vi "Main.vi"(11 "Module Admin":refnum<class "Delacor_lib_QMH_Module Admin.lvclass">) -> ()   [LabVIEW 2019, in "Main UI.lvlib"]
doc: "This template is based off of the Queued Message Handler design pattern and the Queued Message Handler project template that ships with LabVIEW.\n\nThe main difference is that the queue is private to this module and communication between modules is performed via Broadcast and Request events.\n\nRequest events are wrapped in public API methods and are handled in the Event Handling Loop (EHL) of this VI. Any module can register for Broadcast events sent by this module. The EHL generates messages based on user interface actions.\n\nThe Message Handling Loop (MHL) processes messages generated by the EHL, or by other messages. The messages are string values, so new messages can be added easily to the Message Cases case structure in the MHL. Each message cluster can also provide an optional value for Message Data, which is a variant that can be converted to whatever message-specific data is required.\n_____\nBased on Delacor QMH Project Template 4.0.0.47.\n_____\nBased on DQMH Project Template 6.1.0.94."
uses:
  Main UI.lvlib
  <vilib>/Delacor/Delacor QMH/Libraries/Module Admin_class/Delacor_lib_QMH_Module Admin.lvclass
  Main UI Shared/Decimation input --cluster.ctl
  Neo-Laura-LVOOP/Class Library/XYgraph_class/Units --enum.ctl
  Main UI Shared/Zpos type.ctl
  Main UI Shared/Apply_Savitsky--cluster.ctl
  FileReader/FPref_clustered--cluster references.ctl
  Main UI Shared/Boolean--FP cluster.ctl
  FileReader/FPref_cntrls--cluster references.ctl
  Main UI Shared/Indicators--FP cluster.ctl
  Module Data--cluster.ctl
  Neo-Laura-LVOOP/Class Library/XYgraph_class/XYgraph.lvclass
  <vilib>/Delacor/Delacor QMH/Libraries/Message Queue_class/Delacor_lib_QMH_Message Queue.lvclass/Delacor_lib_QMH_Message Queue.ctl
  <vilib>/event_ctls.llb/lveventtype.ctl
  Get analysis parameters Argument--cluster.ctl
  Get analysis parameters (Reply Payload)--cluster.ctl
  Stop Argument--cluster.ctl
  Filepath updated Argument--cluster.ctl
  Filepath Editor/Settings--cluster.ctl
  <vilib>/Delacor/Delacor QMH/Libraries/Module Admin_class/Delacor_lib_QMH_Module Admin.lvclass/Delacor_lib_QMH_Module Admin.ctl
  <vilib>/Delacor/Delacor QMH/Libraries/Message Queue_class/Delacor_lib_QMH_Enqueue Message (Single).vi
  <vilib>/Delacor/Delacor QMH/Libraries/Module Admin_class/Delacor_lib_QMH_Get External Launch.vi
  <vilib>/Utility/error.llb/Error Cluster From Error Code.vi
  <vilib>/ErrorRing/Error Ring.xnode
  <vilib>/Delacor/Delacor QMH/Libraries/Message Queue_class/Delacor_lib_QMH_Message Queue.lvclass
  Filepath Editor/Filepath Editor.lvlib
  Analysis/Analysis.lvlib
  FileReader/FileReader.lvlib
  Main UI Shared/MAIN UI Shared.lvlib
panel:
  out "XYgraph":cluster{"X":dbl[], "Y":dbl[]}[](graph)
  out "FileReader Running?":bool
  out "Settings Editor Running?":bool
  out "Analysis Running?":bool
  in  "Apply savitzky":T1
  in  "File number":i16=-21550 min=-1 max=1 step=1
  in  "Live?":bool
  in  "Z pos (ch)":T2 items=["Sensor FB", "Virtual"]
  in  "Tau Delay (ms)":dbl
  in  "Contact":T3={"Contact stat?"=TRUE, "Contact Spread of dev"=0.0} {"Contact Spread of dev" format="%#_13g"}
  out "Status":string
  in  "Y Units (micro)":T4="pico"
  in  "X Units (micro)":T4="micro"
  out "Files in Directory":i16=-21550
  out "Size (bytes)":i64=37399506 format="%.0p"
  in  "Savitzksky-Golay":T5={"Sidepoints (M)"=20.0, "Filter Order"=5} {"Filter Order" scale=0.0..10.0; "Sidepoints (M)" scale=0.0..10.0}
  out "Fcurve Metadata":string[][](table)
  in  "Decimation":T6={"App"={"Dec"=1, "apply"=FALSE}, "Con"={"Dec"=1, "apply"=FALSE}, "Ret"={"Dec"=1, "apply"=FALSE}}
  in  "Fwd":bool
  in  "Prev":bool
  in  "Settings":bool
  in  "Load":bool
  out "Filepath":path
  out "error out":errorcluster
  out "version":string
  # "TDMS file viewer"
  # "Def"
  # "Zpos"
  # "Contact"
  # "Analysis Parameters"
  # "Metadata"
  # "Decimation"
  # "Savitzsky-Golay Parameters"
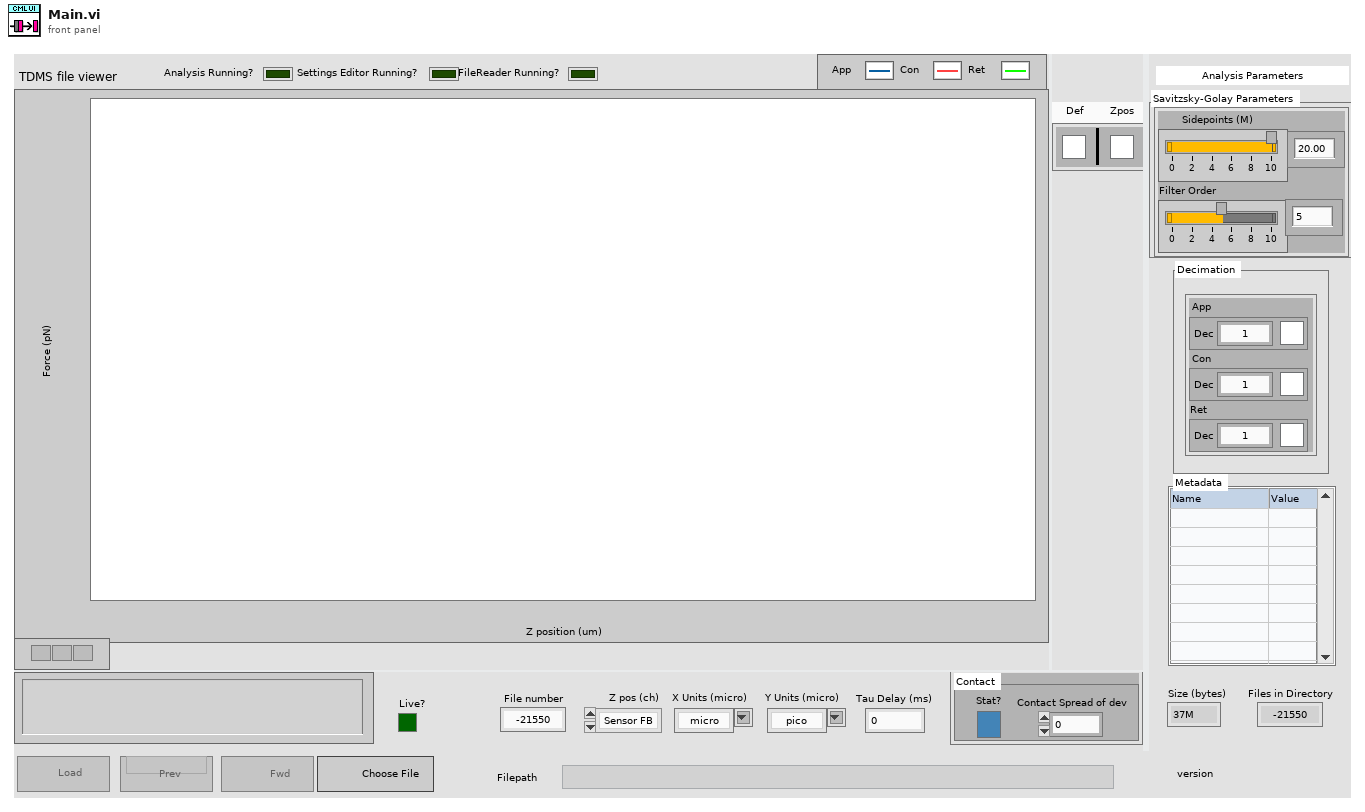
[diagram p1: front panel]
types:
  T1 = typedef "MAIN UI Shared.lvlib/Apply_Savitsky--cluster.ctl" = cluster{"Def":bool, "Zpos":bool}
  T2 = typedef "MAIN UI Shared.lvlib/Zpos type.ctl" = u16
  T3 = cluster{"Contact stat?":bool, "Contact Spread of dev":dbl}
  T4 = typedef "XYgraph.lvclass/Units --enum.ctl" = string
  T5 = cluster{"Sidepoints (M)":dbl, "Filter Order":i32}
  T6 = typedef "MAIN UI Shared.lvlib/Decimation input --cluster.ctl" = cluster{"App":cluster{"Dec":i32, "apply":bool}, "Con":cluster{"Dec":i32, "apply":bool}, "Ret":cluster{"Dec":i32, "apply":bool}}
  T7 = typedef "Indicators--FP cluster.ctl" = cluster{"Fcurve Metadata":refnum<vi>, "XYgraph":refnum<vi>, "Size (bytes)":refnum<vi>, "Files in Directory":refnum<vi>, "Filepath":refnum<vi>}
  T8 = typedef "FPref_clustered--cluster references.ctl" = cluster{" bools":T9, "cntrls":T10, "Ind":T7}
  T9 = typedef "MAIN UI Shared.lvlib/Boolean--FP cluster.ctl" = cluster{"Load":refnum<vi>, "Prev":refnum<vi>, "Fwd":refnum<vi>, "Set filepath":refnum<vi>}
  T10 = typedef "FPref_cntrls--cluster references.ctl" = cluster{"Z pos (ch)":refnum<vi>, "Tau Delay (ms)":refnum<vi>, "Y Units (micro)":refnum<vi>, "X Units (micro)":refnum<vi>, "Contact Spread of dev":refnum<vi>, "Contact stat?":refnum<vi>, "Decimation":refnum<vi>, "Savitzksky-Golay":refnum<vi>, "Apply savitzky ":refnum<vi>, "File number":refnum<vi>}
  T11 = cluster{"Fcurve Metadata":refnum<vi>, "XYgraph":refnum<vi>, "Size (bytes)":refnum<vi>, "Files in Directory":refnum<vi>, "Filepath":refnum<vi>}
  T12 = cluster{"Z pos (ch)":refnum<vi>, "Tau Delay (ms)":refnum<vi>, "Y Units (micro)":refnum<vi>, "X Units (micro)":refnum<vi>, "Contact Spread of dev":refnum<vi>, "Contact stat?":refnum<vi>, "Decimation":refnum<vi>, "Savitzksky-Golay":refnum<vi>, "Apply savitzky ":refnum<vi>, "File number":refnum<vi>}
  T13 = cluster{"Load":refnum<vi>, "Prev":refnum<vi>, "Fwd":refnum<vi>, "Set file path":refnum<vi>}
  T14 = typedef "Main UI.lvlib/Request Events--cluster.ctl" = cluster{"Stop Module":refnum<user-event>, "Show Panel":refnum<user-event>, "Hide Panel":refnum<user-event>, "Get Module Execution Status":refnum<user-event>, "Show Diagram":refnum<user-event>, "Get analysis parameters":refnum<user-event>, "Filepath updated":refnum<user-event>}
  T15 = typedef "Filepath Editor.lvlib/Broadcast Events--cluster.ctl" = cluster{"Module Did Init":refnum<user-event>, "Status Updated":refnum<user-event>, "Error Reported":refnum<user-event>, "Module Did Stop":refnum<user-event>, "Update Module Execution Status":refnum<user-event>, "TDMS path settings updated":refnum<user-event>}
  T16 = typedef "Analysis.lvlib/Broadcast Events--cluster.ctl" = cluster{"Module Did Init":refnum<user-event>, "Status Updated":refnum<user-event>, "Error Reported":refnum<user-event>, "Module Did Stop":refnum<user-event>, "Update Module Execution Status":refnum<user-event>, "Fcurve sorted":refnum<user-event>}
  T17 = typedef "FileReader.lvlib/Broadcast Events--cluster.ctl" = cluster{"Module Did Init":refnum<user-event>, "Status Updated":refnum<user-event>, "Error Reported":refnum<user-event>, "Module Did Stop":refnum<user-event>, "Update Module Execution Status":refnum<user-event>}
  T18 = typedef "Main UI.lvlib/Module Data--cluster.ctl" = cluster{"Status":string, "XYgraph Obj":refnum<class "XYgraph.lvclass">, "Ch Datum":waveform(dbl)[], "File loaded":bool, "FPref":T8, "Tdms filepaths":path[], "TDMS filepath":path}
  T19 = typedef "Main UI.lvlib/Get analysis parameters Argument--cluster.ctl" = cluster{"Wait Notifier":refnum<notifier>, "wait for reply":bool}
  T20 = enum32{"invalid lock state", "Not Locked", "Locked (No Password)", "Password-protected"}
  T21 = typedef "Main UI.lvlib/Stop Argument--cluster.ctl" = cluster{"Origin":string, "Exit via Stop Module Req?":bool, "Wait for Module to stop?":bool}
  T22 = typedef "Main UI.lvlib/Filepath updated Argument--cluster.ctl" = cluster{"Settings":T23}
  T23 = typedef "Filepath Editor.lvlib/Settings--cluster.ctl" = cluster{"TDMS Filepath":path, "TDMS Directory":path, "Dir?":bool}
  T24 = enum32{"Invalid", "Standard", "Closed", "Hidden", "Minimized", "Maximized"}
  T25 = cluster{"Contact stat?":bool, "Contact Spread of dev":bool}
  T26 = typedef "lveventtype.ctl" = enum32{"Null", "Timeout", "Annotation Menu Selection", "Annotation Menu Selection?", "App Instance Close", "App Instance Close?", "Autoscale Range Change", "Bookmark Info Change", "Cell Edit", "Cell Edit?", "Cursor Grab", "Cursor Grab?", "Cursor Menu Selection", "Cursor Menu Selection?", "Cursor Move", "Cursor Release", "Data Change", "Direction Change", "Display State Change", "Drag Ended", "Drag Enter", "Drag Leave", "Drag Over", "Drag Source Update", "Drag Starting", "Drag Starting?", "Drop", "Exec State Change", "Key Down", "Key Down?", "Key Repeat", "Key Repeat?", "Key Up", "Listbox Double Click", "Menu Activation?", "Menu Selection (App)", "Menu Selection? (App)", "Menu Selection (User)", "Mouse Down", "Mouse Down?", "Mouse Enter", "Mouse Leave", "Mouse Move", "Mouse Up", "Mouse Wheel", "NI Security User Change (App)", "Pane Size", "Panel Close", "Panel Close?", "Panel Resize", "Plot Attribute Change", "Scale Range Change", "Shortcut Menu Activation?", "Shortcut Menu Selection (App)", "Shortcut Menu Selection? (App)", "Shortcut Menu Selection (User)", "Tree Double Click", "Tree Drag", "Tree Drag?", "Tree Drop", "Tree Drop?", "Tree Item Close", "Tree Item Close?", "Tree Item Open", "Tree Item Open?", "User Event", "Value Change"}
  T27 = cluster{"App":cluster{"Dec":bool, "apply":bool}, "Con":cluster{"Dec":bool, "apply":bool}, "Ret":cluster{"Dec":bool, "apply":bool}}
  T28 = cluster{"Sidepoints (M)":bool, "Filter Order":bool}
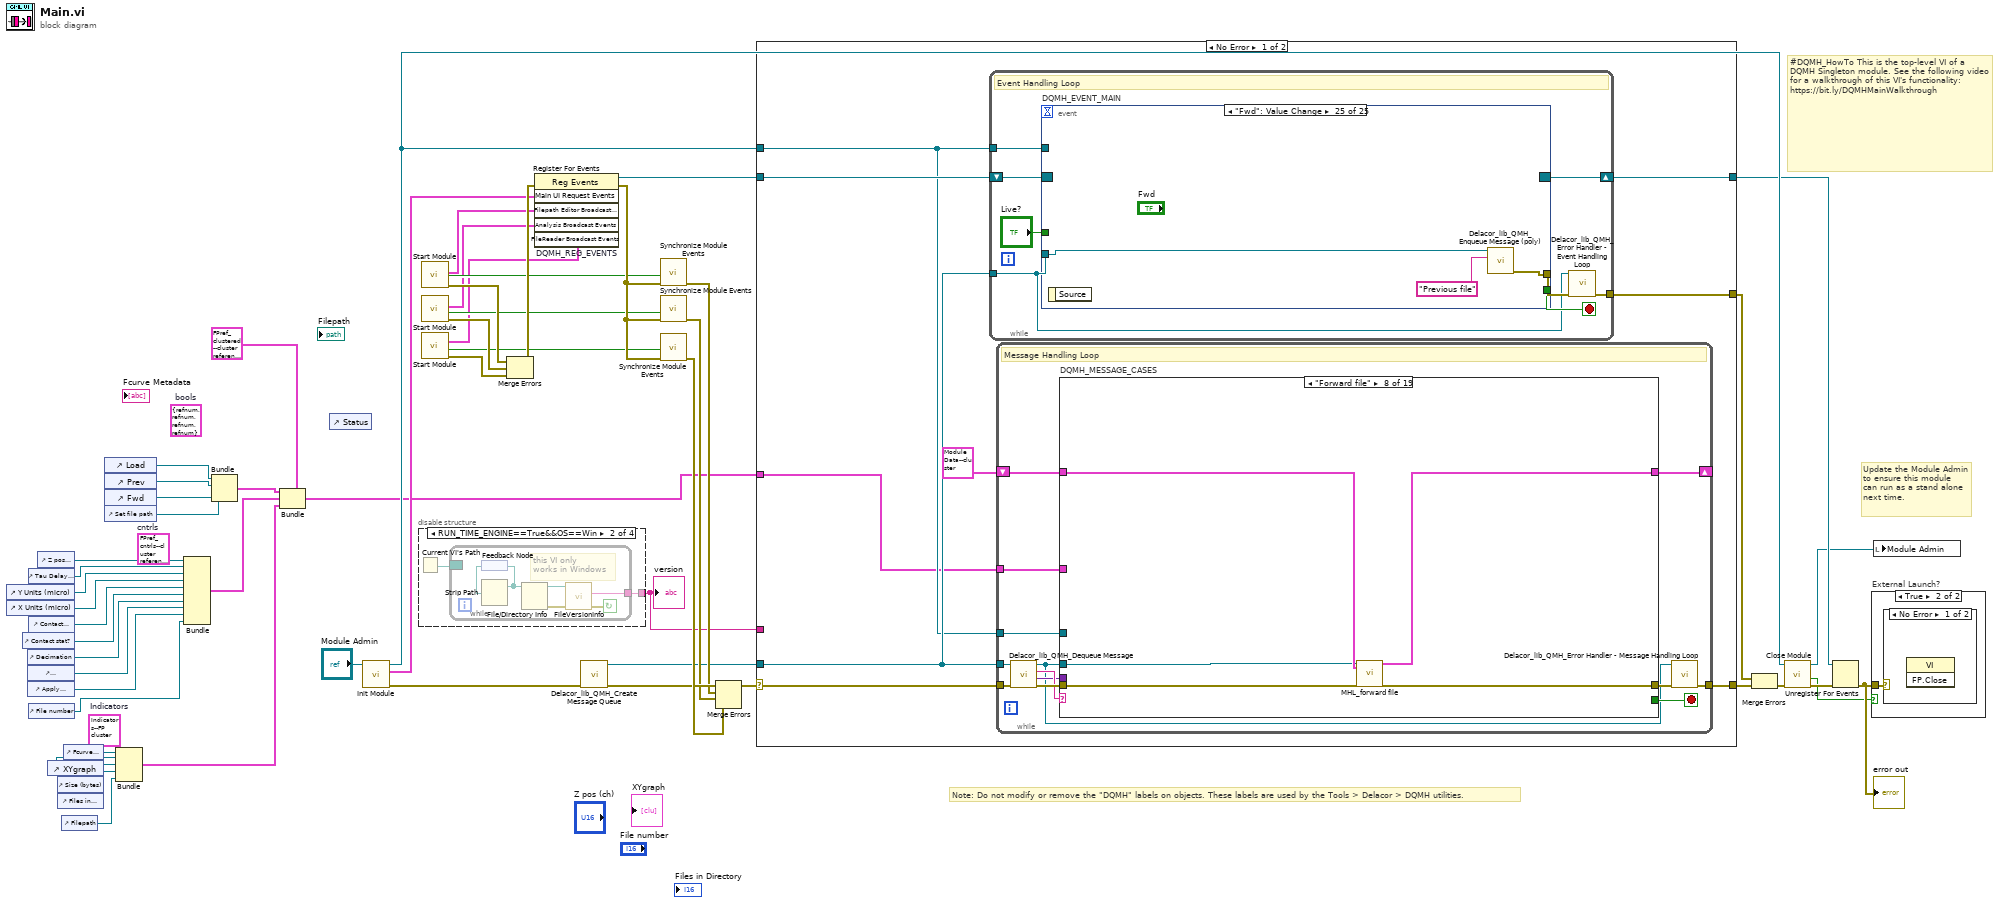
[diagram p0: block diagram]
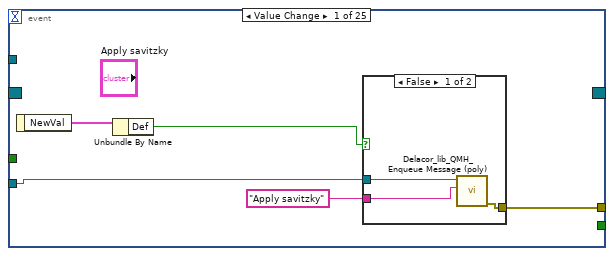
[diagram p2: hidden frame]
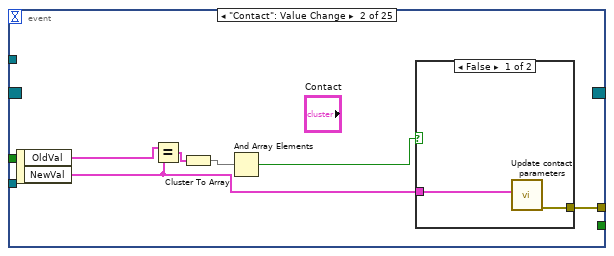
[diagram p4: hidden frame]
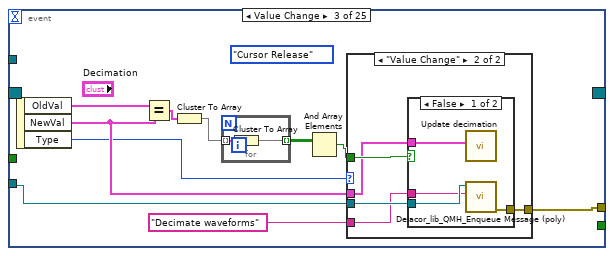
[diagram p6: hidden frame]
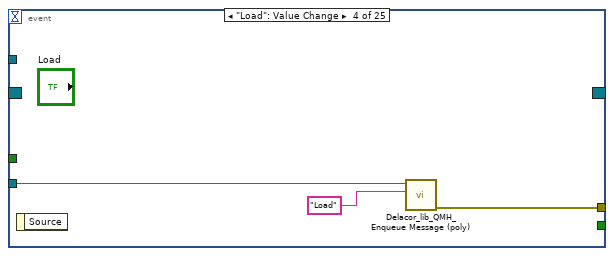
[diagram p9: hidden frame]
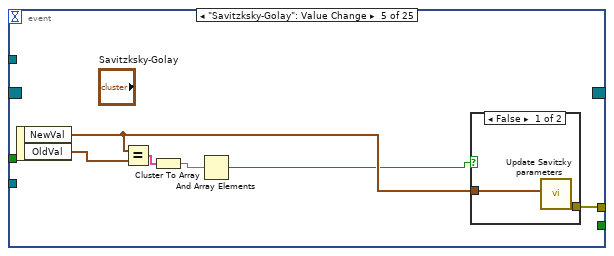
[diagram p10: hidden frame]
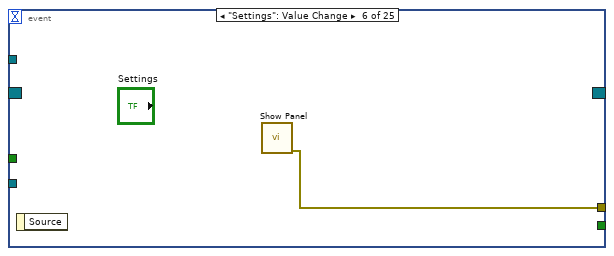
[diagram p12: hidden frame]
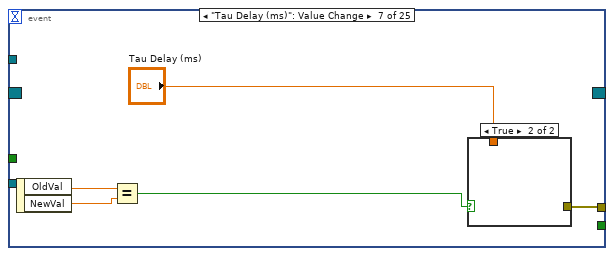
[diagram p13: hidden frame]
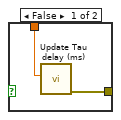
[diagram p14: hidden frame]
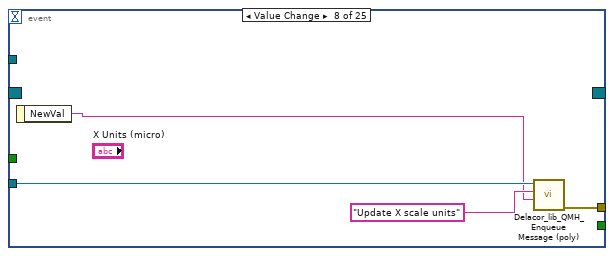
[diagram p15: hidden frame]
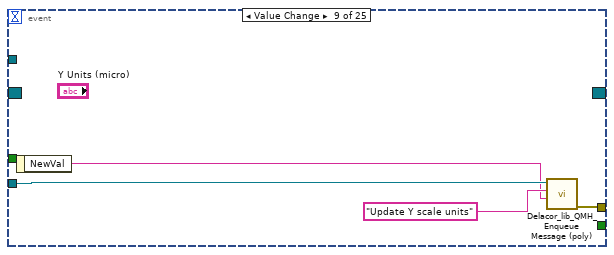
[diagram p16: hidden frame]
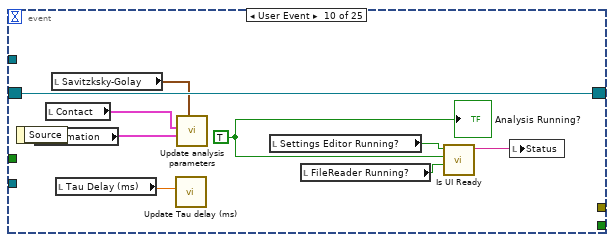
[diagram p17: hidden frame]
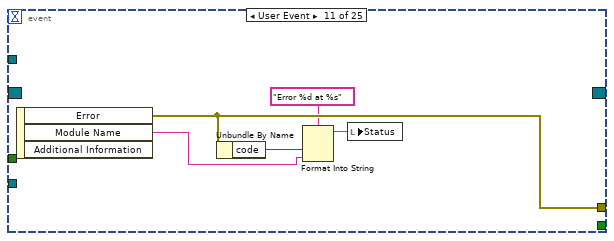
[diagram p18: hidden frame]
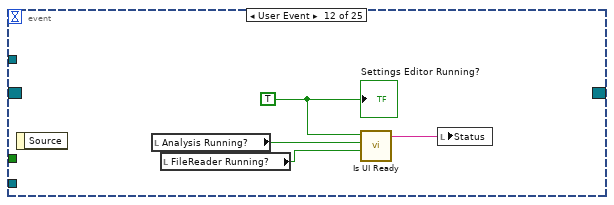
[diagram p19: hidden frame]
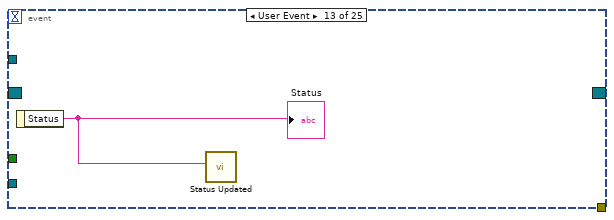
[diagram p20: hidden frame]
diagram:
  (unwired) T7 {"Fcurve Metadata"=refnum, "XYgraph"=refnum, "Size (bytes)"=refnum, "Files in Directory"=refnum, "Filepath"=refnum}  # Indicators
  (unwired) T10 {"Z pos (ch)"=refnum, "Tau Delay (ms)"=refnum, "Y Units (micro)"=refnum, "X Units (micro)"=refnum, "Contact Spread of dev"=refnum, "Contact stat?"=refnum, "Decimation"=refnum, "Savitzksky-Golay"=refnum, "Apply savitzky "=refnum, "File number"=refnum}  # cntrls
  (unwired) T9 {"Load"=refnum, "Prev"=refnum, "Fwd"=refnum, "Set filepath"=refnum}  # bools
  # "#DQMH_HowTo This is the top-level VI of a DQMH Singleton module. See the following video for a walkthrough of this VI's functionality: https://bit.ly/DQMHMainWalkthrough"
  # "Note: Do not modify or remove the \"DQMH\" labels on objects. These labels are used by the Tools > Delacor > DQMH utilities."
  # "Update the Module Admin to ensure this module can run as a stand alone next time."
  n1 = control-ref of="Y Units (micro)"() -> (w18:refnum<vi>)
  n2 = control-ref of="X Units (micro)"() -> (w17:refnum<vi>)
  n3 = control-ref of="Contact stat?"() -> (w15:refnum<vi>)
  n4 = control-ref of="Decimation"() -> (w14:refnum<vi>)
  n5 = control-ref of="Savitzksky-Golay"() -> (w13:refnum<vi>)
  n6 = control-ref of="Apply savitzky"() -> (w12:refnum<vi>)
  n7 = control-ref of="Tau Delay (ms)"() -> (w19:refnum<vi>)
  n8 = control-ref of="Contact Spread of dev"() -> (w16:refnum<vi>)
  n9 = control-ref of="File number"() -> (w2:refnum<vi>)
  n10 = control-ref of="Z pos (ch)"() -> (w20:refnum<vi>)
  n11 = control-ref of="XYgraph"() -> (w6:refnum<vi>)
  n12 = control-ref of="Size (bytes)"() -> (w5:refnum<vi>)
  n13 = control-ref of="Files in Directory"() -> (w4:refnum<vi>)
  n14 = control-ref of="Filepath"() -> (w1:refnum<vi>)
  n15 = control-ref of="Fcurve Metadata"() -> (w7:refnum<vi>)
  n16 = control-ref of="Load"() -> (w21:refnum<vi>)
  n17 = control-ref of="Prev"() -> (w22:refnum<vi>)
  n18 = control-ref of="Fwd"() -> (w23:refnum<vi>)
  n19 = control-ref of="Set file path"() -> (w24:refnum<vi>)
  n20 = Bundle("Fcurve Metadata"=w7, "XYgraph"=w6, "Size (bytes)"=w5, "Files in Directory"=w4, "Filepath"=w1) -> (w3:T11)  [unwired: 1 in]
  n21 = Bundle("Z pos (ch)"=w20, "Tau Delay (ms)"=w19, "Y Units (micro)"=w18, "X Units (micro)"=w17, "Contact Spread of dev"=w16, "Contact stat?"=w15, "Decimation"=w14, "Savitzksky-Golay"=w13, "Apply savitzky"=w12, "File number"=w2) -> (w9:T12)  [unwired: 1 in]
  n22 = Bundle("Load"=w21, "Prev"=w22, "Fwd"=w23, "Set file path"=w24) -> (w10:T13)  [unwired: 1 in]
  n23 = Bundle(cluster=T8 {" bools"={"Load"=refnum, "Prev"=refnum, "Fwd"=refnum, "Set filepath"=refnum}, "cntrls"={"Z pos (ch)"=refnum, "Tau Delay (ms)"=refnum, "Y Units (micro)"=refnum, "X Units (micro)"=refnum, "Contact Spread of dev"=refnum, "Contact stat?"=refnum, "Decimation"=refnum, "Savitzksky-Golay"=refnum, "Apply savitzky "=refnum, "File number"=refnum}, "Ind"={"Fcurve Metadata"=refnum, "XYgraph"=refnum, "Size (bytes)"=refnum, "Files in Directory"=refnum, "Filepath"=refnum}} ("FPref"), "bools"=w10, "cntrls"=w9, "Ind"=w3) -> (w8:T8)
  n24 = control-ref of="Status"() -> ()  [unwired: 1 out]
  n25 = call "Init Module.vi"("Singleton Module Admin in"="Module Admin") -> ("error out"=w53:errorcluster, "Main UI Request Events"=w36:T14, "Singleton Module Admin out"=w39:refnum<class "Delacor_lib_QMH_Module Admin.lvclass">)  [unwired: 8 in]
  n26 = disable-structure "Conditional Disable Structure" shown="RUN_TIME_ENGINE==True&&OS==Win" {
    disable-tunnel: ["development" w57 "Mac" "Linux"] -> w25
    frame condition #0 (active) {
    }
    frame condition #1 {
      n27 = Current VI's Path() -> (path=w58:path)
      n28 = while {
        border: w58 -> [_]
        tunnel: [w59] -> w57
        stop <- w63 continue-if-true
        # "this VI only \nworks in Windows"
        n29 = feedback #1() -> (w62:path)
        n30 = Strip Path(path=w62) -> (stripped path=w61:path)  [unwired: 1 out]
        n31 = feedback-in #1(w61) -> ()
        n32 = File/Directory Info(path=w61) -> (path out=w60:path, error out=w64:errorcluster)  [unwired: 1 in, 5 out]
        n33 = call <vilib>:"FileVersionInfo.vi"("error in (no error)"=w64, "Application Path in"=w60) -> ("error out"=w63:errorcluster, "File Version Info"=w59:string)  [unwired: 6 in, 2 out]
      }
    }
    frame condition #2 {
    }
    frame condition #3 {
    }
  }
  "version" <- w25
  n34 = call "Start Module.vi"() -> ("error out"=w44:errorcluster, "Wait for Event Sync?"=w31:bool, "Filepath Editor Broadcast Events"=w30:T15)  [unwired: 8 in, 1 out]
  n35 = call "Start Module.vi"() -> ("error out"=w43:errorcluster, "Wait for Event Sync?"=w28:bool, "Analysis Broadcast Events"=w29:T16)  [unwired: 8 in, 1 out]
  n36 = call "Start Module.vi"() -> ("error out"=w42:errorcluster, "Wait for Event Sync?"=w26:bool, "FileReader Broadcast Events"=w27:T17)  [unwired: 8 in, 1 out]
  n37 = Merge Errors(w44, w43, w42) -> (w41:errorcluster)
  n38 = register-events "DQMH_REG_EVENTS"(error in=w41, w36, w30, w29, w27) -> (reference out=w37:refnum<event-registration>, error out=w40:errorcluster)  [unwired: 1 in]
  n39 = call <vilib>:"Delacor_lib_QMH_Create Message Queue.vi"("error in"=w53) -> ("error out"=w48:errorcluster, "Message Queue"=w35:refnum<class "Delacor_lib_QMH_Message Queue.lvclass">)  [unwired: 9 in]
  n40 = call "Synchronize Module Events.vi"("error in (no error)"=w40, "Wait for Event Sync?"=w31) -> ("error out"=w46:errorcluster)  [unwired: 9 in]
  n41 = call "Synchronize Module Events.vi"("error in (no error)"=w40, "Wait for Event Sync?"=w28) -> ("error out"=w45:errorcluster)  [unwired: 9 in]
  n42 = call "Synchronize Module Events.vi"("error in (no error)"=w40, "Wait for Event Sync?"=w26) -> ("error out"=w55:errorcluster)  [unwired: 9 in]
  n43 = Merge Errors(w48, w46, w45, w55) -> (w47:errorcluster)
  n44 = case shown="No Error" w47 {
    selector: w47 -> [w73 w408]
    tunnel: [w75 w407] -> w54
    tunnel: [w72 w416] -> w38
    tunnel: w37 -> [w70 w416]
    tunnel: w35 -> [w69 w409]
    tunnel: [w74 _] -> w51
    tunnel: w39 -> [w68 w412]
    tunnel: w25 -> [_ _]
    tunnel: w8 -> [w67 _]
    frame No Error {
      n45 = while {
        tunnel: w69 -> [w77]
        shift-right: [w80] -> w72
        shift-left: w70 -> [w81]
        tunnel: [w82] -> w74
        tunnel: w68 -> [w78]
        stop <- w79 stop-if-true
        # "Event Handling Loop"
        n46 = event "DQMH_EVENT_MAIN" shown="[24] \"Fwd\": Value Change" {
          selector: w81 -> [_ _ _ _ _ _ _ _ _ w156 _ _ _ _ _ _ _ _ _ _ _ _ _ _ _]
          dyn-events: [_ _ _ _ _ _ _ _ _ w156 _ _ _ _ _ _ _ _ _ _ _ _ _ _ _] -> w80
          timeout: _ -> [_ _ _ _ _ _ _ _ _ _ _ _ _ _ _ _ _ _ _ _ _ _ _ _ _]
          tunnel: [_ _ _ _ _ _ _ _ _ _ _ _ _ _ _ _ _ _ _ _ TRUE ("Discard?") _ _ _ _] -> w79
          tunnel: w77 -> [w85 _ w101 w121 _ _ _ w141 w146 _ _ _ _ _ _ w180 _ _ _ _ w203 w210 w218 w220 w223]
          tunnel: [w86 w93 w109 w123 w129 w132 w135 w142 w145 _ w161 _ _ w168 _ w174 w182 _ _ _ w206 w212 w213 w219 w222] -> w83
          tunnel: w78 -> [_ _ _ _ _ _ _ _ _ _ _ _ _ _ _ _ _ _ _ _ _ _ _ _ _]
          tunnel: "Live?" -> [_ _ _ _ _ _ _ _ _ _ _ _ _ _ _ _ _ _ _ _ _ _ _ _ _]
          event Value Change {
            n47 = event-data() -> ("NewVal"=w88:T1)  [unwired: 1 in]
            n48 = Unbundle By Name(w88) -> ("Def"=w87:bool)
            n49 = case shown="False" w87 {
              tunnel: [w91 _] -> w86
              tunnel: w85 -> [w90 _]
              tunnel: "Apply savitzky" ("Message") -> [w89 _]
              frame False {
                n50 = call-poly <vilib>:"Delacor_lib_QMH_Enqueue Message (poly).vi"("Message"=w89, "Message Queue in"=w90) -> ("error out"=w91:errorcluster)  [unwired: 8 in, 1 out]
              }
              frame True {
              }
            }
          }
          event "Contact": Value Change {
            n51 = event-data() -> ("OldVal"=w95:T3, "NewVal"=w92:T3)  [unwired: 1 in]
            n52 = Equal?(x=w95, y=w92) -> (x = y?=w97:T25)
            n53 = Cluster To Array(cluster=w97) -> (array=w96:bool[])
            n54 = And Array Elements(Boolean array=w96) -> (logical AND=w94:bool)
            n55 = case shown="False" w94 {
              tunnel: [w99 _] -> w93
              tunnel: w92 -> [w98 _]
              frame False {
                n56 = call "Update contact parameters.vi"("Contact"=w98) -> ("error out"=w99:errorcluster)  [unwired: 10 in]
              }
              frame True {
              }
            }
          }
          event Value Change {
            (unwired) lveventtype."Cursor Release" ("Type")
            n57 = event-data() -> ("OldVal"=w107:T6, "NewVal"=w103:T6, "Type"=w102:T26)  [unwired: 1 in]
            n58 = Equal?(x=w107, y=w103) -> (x = y?=w108:T27)
            n59 = Cluster To Array(cluster=w108) -> (array=w106:cluster{"Dec":bool, "apply":bool}[])
            n60 = for {
              tunnel: w106 -> [w120] mode=indexing
              tunnel: [w119] -> w105 mode=indexing
              n61 = Cluster To Array(cluster=w120) -> (array=w119:bool[])
            }
            n62 = And Array Elements(Boolean array=w105) -> (logical AND=w104:bool)
            n63 = case shown="\"Value Change\"" w102 {
              tunnel: [_ w113] -> w109
              tunnel: w104 -> [_ w114]
              tunnel: w103 -> [_ w110]
              tunnel: w101 -> [_ w112]
              tunnel: "Decimate waveforms" ("Message") -> [_ w111]
              frame "Null", Default {
              }
              frame "Value Change" {
                n64 = case shown="False" w114 {
                  tunnel: [w118 _] -> w113
                  tunnel: w112 -> [w117 _]
                  tunnel: w111 -> [w116 _]
                  tunnel: w110 -> [w115 _]
                  frame False {
                    n65 = call "Update decimation.vi"("Decimation"=w115) -> ()  [unwired: 10 in, 1 out]
                    n66 = call-poly <vilib>:"Delacor_lib_QMH_Enqueue Message (poly).vi"("Message"=w116, "Message Queue in"=w117) -> ("error out"=w118:errorcluster)  [unwired: 8 in, 1 out]
                  }
                  frame True {
                  }
                }
              }
            }
          }
          event "Load": Value Change {
            n67 = event-data() -> ()  [unwired: 1 in, 1 out]
            n68 = call-poly <vilib>:"Delacor_lib_QMH_Enqueue Message (poly).vi"("Message"="Load", "Message Queue in"=w121) -> ("error out"=w123:errorcluster)  [unwired: 8 in, 1 out]
          }
          event "Savitzksky-Golay": Value Change {
            n69 = event-data() -> ("NewVal"=w128:T5, "OldVal"=w127:T5)  [unwired: 1 in]
            n70 = Equal?(x=w128, y=w127) -> (x = y?=w126:T28)
            n71 = Cluster To Array(cluster=w126) -> (array=w125:bool[])
            n72 = And Array Elements(Boolean array=w125) -> (logical AND=w124:bool)
            n73 = case shown="False" w124 {
              tunnel: [w131 _] -> w129
              tunnel: w128 -> [w130 _]
              frame False {
                n74 = call "Update Savitzky parameters.vi"("Savitzksky-Golay"=w130) -> ("error out"=w131:errorcluster)  [unwired: 10 in]
              }
              frame True {
                # "Dont \nupdate"
              }
            }
          }
          event "Settings": Value Change {
            n75 = event-data() -> ()  [unwired: 1 in, 1 out]
            n76 = call "Show Panel.vi"() -> ("error out"=w132:errorcluster)  [unwired: 11 in]
          }
          event "Tau Delay (ms)": Value Change {
            n77 = event-data() -> ("OldVal"=w137:dbl, "NewVal"=w136:dbl)  [unwired: 1 in]
            n78 = Equal?(x=w137, y=w136) -> (x = y?=w134:bool)
            n79 = case shown="True" w134 {
              tunnel: [w139 _] -> w135
              tunnel: "Tau Delay (ms)" -> [w138 _]
              frame False {
                n80 = call "Update Tau delay (ms).vi"("Tau Delay (ms)"=w138) -> ("error out"=w139:errorcluster)  [unwired: 10 in]
              }
              frame True {
              }
            }
          }
          event Value Change {
            n81 = event-data() -> ("NewVal"=w140:T4)  [unwired: 1 in]
            n82 = call-poly <vilib>:"Delacor_lib_QMH_Enqueue Message (poly).vi"("Message Data"=w140, "Message"="Update X scale units", "Message Queue in"=w141) -> ("error out"=w142:errorcluster)  [unwired: 7 in, 1 out]
          }
          event Value Change {
            n83 = event-data() -> ("NewVal"=w144:T4)  [unwired: 1 in]
            n84 = call-poly <vilib>:"Delacor_lib_QMH_Enqueue Message (poly).vi"("Message Data"=w144, "Message"="Update Y scale units", "Message Queue in"=w146) -> ("error out"=w145:errorcluster)  [unwired: 7 in, 1 out]
          }
          event User Event {
            w154 = TRUE ("Acquisition Running?")
            n85 = event-data() -> ()  [unwired: 1 in, 1 out]
            n86 = local read "Decimation"() -> (w150:T6)
            n87 = local read "Contact"() -> (w149:T3)
            n88 = local read "Savitzksky-Golay"() -> (w151:T5)
            n89 = local read "Tau Delay (ms)"() -> (w148:dbl)
            n90 = call "Update Tau delay (ms).vi"("Tau Delay (ms)"=w148) -> ()  [unwired: 10 in, 1 out]
            n91 = call "Update analysis parameters.vi"("Savitzksky-Golay"=w151, "Decimation"=w150, "Contact"=w149) -> ()  [unwired: 6 in, 3 out]
            n92 = local read "Settings Editor Running?"() -> (w153:bool)
            n93 = local read "FileReader Running?"() -> (w152:bool)
            n94 = call "Is UI Ready.vi"("Logger Running?"=w152, "Acquisition Running?"=w154, "Settings Editor Running?"=w153) -> ("Status"=w155:string)  [unwired: 8 in]
            n95 = local write "Status"(w155) -> ()
            "Analysis Running?" <- w154
          }
          event User Event {
            n96 = event-data() -> ("Error"=w161:errorcluster, "Module Name"=w159:string)  [unwired: 1 in, 1 out]
            n97 = Unbundle By Name(w161) -> ("code"=w160:i32)
            n98 = Format Into String(format string="Error %d at %s", w160, w159) -> (resulting string=w158:string)  [unwired: 2 in, 1 out]
            n99 = local write "Status"(w158) -> ()
          }
          event User Event {
            w163 = TRUE ("Settings Editor Running?")
            n100 = event-data() -> ()  [unwired: 1 in, 1 out]
            n101 = local read "Analysis Running?"() -> (w165:bool)
            n102 = local read "FileReader Running?"() -> (w164:bool)
            n103 = call "Is UI Ready.vi"("Logger Running?"=w164, "Acquisition Running?"=w165, "Settings Editor Running?"=w163) -> ("Status"=w162:string)  [unwired: 8 in]
            n104 = local write "Status"(w162) -> ()
            "Settings Editor Running?" <- w163
          }
          event User Event {
            n105 = event-data() -> ("Status"=w166:string)  [unwired: 1 in]
            "Status" <- w166
            n106 = call "Status Updated.vi"("Status"=w166) -> ()  [unwired: 10 in, 1 out]
          }
          event User Event {
            n107 = event-data() -> ("Settings"=w167:T23)  [unwired: 1 in]
            n108 = Unbundle By Name(w167) -> ("TDMS Filepath"=w169:path)
            n109 = local write "Filepath"(w169) -> ()
            n110 = call "Filepath updated.vi"("Settings"=w167) -> ("error out"=w168:errorcluster)  [unwired: 10 in]
          }
          event User Event {
            w172 = TRUE ("Logger Running?")
            n111 = event-data() -> ()  [unwired: 1 in, 1 out]
            n112 = local read "Settings Editor Running?"() -> (w171:bool)
            n113 = local read "Analysis Running?"() -> (w170:bool)
            n114 = call "Is UI Ready.vi"("Logger Running?"=w172, "Acquisition Running?"=w170, "Settings Editor Running?"=w171) -> ("Status"=w173:string)  [unwired: 8 in]
            n115 = local write "Status"(w173) -> ()
            "FileReader Running?" <- w172
          }
          event User Event {
            # "Another Module called the \"Get analysis parameters\" API Method."
            n116 = event-data() -> ("Wait Notifier"=w176:refnum<notifier>, "wait for reply"=w175:bool)  [unwired: 1 in]
            n117 = Bundle(cluster=T19 {"Wait Notifier"=refnum, "wait for reply"=FALSE} ("Get analysis parameters Argument"), "Wait Notifier"=w176, "wait for reply"=w175) -> (w177:T19)
            n118 = call-poly <vilib>:"Delacor_lib_QMH_Enqueue Message (poly).vi"("Message Data"=w177, "Message"="Get analysis parameters", "Message Queue in"=w180) -> ("error out"=w174:errorcluster)  [unwired: 7 in, 1 out]
          }
          event User Event {
            # "Another Module called the \"Get Module Execution Status\" API Method."
            n119 = event-data() -> ()  [unwired: 1 in, 1 out]
            n120 = call "Update Module Execution Status.vi"("Running?"=TRUE) -> ("error out"=w182:errorcluster)  [unwired: 10 in]
          }
          event User Event {
            # "Hide the panel of this VI, and send a status updated message to let listeners know."
            # "Another Module called the \"Hide Panel\" API Method."
            n121 = event-data() -> ()  [unwired: 1 in, 1 out]
            n122 = control-ref of="This VI"() -> (w184:refnum<vi>)
            n123 = call "Hide VI Panel.vi"("VI"=w184) -> ()  [unwired: 10 in, 1 out]
            n124 = call "Status Updated.vi"("Status"="Panel hidden." ("format string")) -> ()  [unwired: 10 in, 1 out]
          }
          event User Event {
            # "Another Module called the \"Show Diagram\" API Method. This event is used for debugging."
            n125 = event-data() -> ()  [unwired: 1 in, 1 out]
            n126 = disable-structure shown="RUN_TIME_ENGINE==False" {
              frame condition #0 (active) {
                # "functionality not available in exe"
                n127 = invoke on="Invoke Node" class="VI" method="Lock State.Get"() -> (error out=w190:errorcluster, "Get Lock State"=w189:T20, "pwd in cache"=w186:bool)  [unwired: 4 in, 1 out]
                n128 = Equal?(x=T20."Password-protected", y=w189) -> (x = y?=w187:bool)
                n129 = Compound Arithmetic op=AND(w187, invert w186) -> (w185:bool)
                n130 = case shown="False" w185 {
                  tunnel: w190 -> [w193 _]
                  frame False {
                    n131 = property on="Property Node" class="VI"(error in=w193, "BDWin.Open"=TRUE ("Block Diagram Window:Open")) -> ()  [unwired: 1 in, 2 out]
                    n132 = call "Status Updated.vi"("Status"="Block Diagram shown." ("format string")) -> ()  [unwired: 10 in, 1 out]
                  }
                  frame True {
                    # "Password-protected VI, and the password is not in the cache. Do not show the diagram."
                  }
                }
              }
              frame condition #1 {
              }
            }
          }
          event User Event {
            # "Show the panel of this VI, and send a status updated message to let listeners know."
            # "Another Module called the \"Show Panel\" API Method."
            n133 = event-data() -> ()  [unwired: 1 in, 1 out]
            n134 = control-ref of="This VI"() -> (w195:refnum<vi>)
            n135 = call "Open VI Panel.vi"("VI"=w195) -> ()  [unwired: 10 in, 1 out]
            n136 = call "Status Updated.vi"("Status"="Panel shown." ("format string")) -> ()  [unwired: 10 in, 1 out]
          }
          event User Event {
            # "The Stop Module Event can get fired from the Exit message in the MHL. The queue gets destroyed in that case. If the queue no longer exists, the Enqueue Exit as a priority message will return error 1. It is safe to ignore, because the module is already exiting."
            # "Another Module called the \"Stop Module\" API Method  or the Message Handling Loop below."
            n137 = event-data() -> ("Origin"=w202:string, "Exit via Stop Module Req?"=w198:bool, "Wait for Module to stop?"=w197:bool)  [unwired: 1 in]
            n138 = local write "Status"(w202) -> ()
            n139 = Bundle By Name(cluster=T21 {"Origin"="", "Exit via Stop Module Req?"=FALSE, "Wait for Module to stop?"=FALSE} ("Stop Argument"), "Exit via Stop Module Req?"=w198, "Wait for Module to stop?"=w197) -> (w196:T21)
            n140 = call-poly <vilib>:"Delacor_lib_QMH_Enqueue Message (poly).vi"("Priority Message? (F)"=TRUE, "Message Data"=w196, "Message"="Exit", "Message Queue in"=w203) -> ("error out"=w207:errorcluster)  [unwired: 6 in, 1 out]
            n141 = call <vilib>:"Clear Errors.vi"("error in (no error)"=w207, "specific error code to clear (0: all)"=1) -> ("error out"=w206:errorcluster)  [unwired: 4 in, 1 out]
          }
          event Panel Close? {
            w211 = TRUE  # Discard the event, the MHL is responsible for closing and stopping this VI.
            # "this is the top level application, it always exits"
            # "Hide the panel or send the 'Exit' message if the user clicks the 'X' on the module main VI panel."
            n142 = event-data() -> ()  [unwired: 1 in, 1 out]
            n143 = call-poly <vilib>:"Delacor_lib_QMH_Enqueue Message (poly).vi"("Priority Message? (F)"=TRUE, "Message"="Exit", "Message Queue in"=w210) -> ("error out"=w212:errorcluster)  [unwired: 7 in, 1 out]
            n144 = event-data ("Event Filter Node")("Discard?"=w211) -> ()  [unwired: 1 in, 1 out]
          }
          event User Event {
            # "Another Module called the \"Filepath updated\" API Method."
            n145 = event-data() -> ("Settings"=w214:T23)  [unwired: 1 in]
            n146 = Bundle(cluster=T22 {"Settings"={"TDMS Filepath"=path "", "TDMS Directory"=path "", "Dir?"=FALSE}} ("Filepath updated Argument"), "Settings"=w214) -> (w215:T22)
            n147 = call-poly <vilib>:"Delacor_lib_QMH_Enqueue Message (poly).vi"("Message Data"=w215, "Message"="Filepath updated", "Message Queue in"=w218) -> ("error out"=w213:errorcluster)  [unwired: 7 in, 1 out]
          }
          event "Prev": Value Change {
            n148 = event-data() -> ()  [unwired: 1 in, 1 out]
            n149 = call-poly <vilib>:"Delacor_lib_QMH_Enqueue Message (poly).vi"("Message"="Previous file", "Message Queue in"=w220) -> ("error out"=w219:errorcluster)  [unwired: 8 in, 1 out]
          }
          event "Fwd": Value Change {
            n150 = event-data() -> ()  [unwired: 1 in, 1 out]
            n151 = call-poly <vilib>:"Delacor_lib_QMH_Enqueue Message (poly).vi"("Message"="Previous file", "Message Queue in"=w223) -> ("error out"=w222:errorcluster)  [unwired: 8 in, 1 out]
          }
        }
        n152 = call-dynamic "Delacor_lib_QMH_Error Handler - Event Handling Loop.vi"("error in"=w83, "Message Queue in"=w77) -> ("dup error in"=w82:errorcluster)  [unwired: 8 in, 1 out]
      }
      n153 = while {
        tunnel: w69 -> [w228]
        shift-right: [w232] -> _
        shift-left: T18 {"Status"="", "XYgraph Obj"=refnum, "Ch Datum"=[], "File loaded"=FALSE, "FPref"={" bools"={"Load"=refnum, "Prev"=refnum, "Fwd"=refnum, "Set filepath"=refnum}, "cntrls"={"Z pos (ch)"=refnum, "Tau Delay (ms)"=refnum, "Y Units (micro)"=refnum, "X Units (micro)"=refnum, "Contact Spread of dev"=refnum, "Contact stat?"=refnum, "Decimation"=refnum, "Savitzksky-Golay"=refnum, "Apply savitzky "=refnum, "File number"=refnum}, "Ind"={"Fcurve Metadata"=refnum, "XYgraph"=refnum, "Size (bytes)"=refnum, "Files in Directory"=refnum, "Filepath"=refnum}}, "Tdms filepaths"=[], "TDMS filepath"=path ""} ("Data Cluster") -> [w233]
        tunnel: w73 -> [w236]
        tunnel: [w234] -> w75
        tunnel: w68 -> [w226]
        tunnel: w67 -> [w225]
        stop <- w231 stop-if-true
        # "Message Handling Loop"
        n154 = call-dynamic "Delacor_lib_QMH_Dequeue Message.vi"("error in"=w236, "Message Queue in"=w228) -> ("error out"=w235:errorcluster, "Message Data"=w229:variant, "Message"=w230:string, "Message Queue out"=w227:refnum<class "Delacor_lib_QMH_Message Queue.lvclass">)  [unwired: 6 in]
        n155 = case "DQMH_MESSAGE_CASES" shown="\"Forward file\"" w230 {
          selector: w230 -> [_ _ _ _ _ _ _ _ _ _ _ _ _ _ _ _ _ _ w394]
          tunnel: w227 -> [_ _ _ _ _ _ w305 w310 _ _ w325 _ _ _ _ _ w358 w385 _]
          tunnel: w235 -> [w265 w269 w274 w279 w293 w304 w309 w314 w322 w324 w334 w337 w341 w344 w353 w355 w365 w390 w396]
          tunnel: [w263 w269 w273 w282 w296 w304 w308 w313 w317 w324 w326 w336 w338 w345 w352 w355 w361 w374 w397] -> w237
          tunnel: w233 -> [w254 w268 w272 w281 w295 w303 w307 w312 w316 w323 w330 w335 w340 w343 w351 w354 w360 w384 w395]
          tunnel: [w249 w268 w270 w280 w294 w303 w306 w311 w315 w323 w329 w335 w339 w342 w351 w354 w360 w384 w395] -> w232
          tunnel: [_ _ _ _ _ _ _ _ _ _ _ _ _ _ _ _ _ w383 _] -> w231
          tunnel: w229 -> [_ _ _ w276 w290 _ _ _ w320 _ w333 _ _ _ _ _ w359 w382 _]
          tunnel: w226 -> [w255 _ _ _ _ _ _ _ _ _ _ _ _ _ _ _ w357 w377 _]
          tunnel: w225 -> [w238 _ _ _ _ _ _ _ _ _ _ _ _ _ _ _ _ _ _]
          frame "Initialize" {
            (unwired) cluster{"X":dbl[], "Y":dbl[]}[] [] ("Data")
            w250 = "Initial Message" ("Initial Message")
            # "Enable: Start, Settings\nDisable: Stop"
            # "Initialize - Any operation that needs to be done before the module can receive messages. Synchronize Caller Events.vi will inform Start Module.vi that the module has launched and is ready to receive messages. Module Did Init.vi will broadcast that the module initialized."
            n156 = control-ref of="XYgraph"() -> (w241:refnum<vi>)
            n157 = call "Synchronize Caller Events.vi"("error in (no error)"=w265, "Singleton Module Admin in"=w255) -> ("error out"=w264:errorcluster, "Singleton Module Admin out"=w251:refnum<class "Delacor_lib_QMH_Module Admin.lvclass">)  [unwired: 8 in]
            n158 = Unbundle By Name(w238) -> ("bools"=w239:T9)
            n159 = property on="Property Node" class="Module Admin"(reference=w251) -> ("Accessors:External Launch"=w259:bool)  [unwired: 1 in, 2 out]
            n160 = call "XYgraph_Create.vi"("FPref"=w241) -> ("reference out"=w240:refnum<class "XYgraph.lvclass">)  [unwired: 17 in, 1 out]
            n161 = Select(t=T24."Hidden" ("State"), s=w259, f=T24."Standard" ("State")) -> (s? t:f=w256:T24)
            n162 = call "Module Name--constant.vi"() -> ("Module Name"=w262:string)  [unwired: 11 in]
            n163 = Bundle By Name(cluster=w254, "Status"=w250, "XYgraph Obj"=w240, "FPref"=w238) -> (w249:T18)
            n164 = property on="Property Node" class="VI"("Front Panel.Title"=w262) -> (reference out=w261:refnum<vi>, error out=w267:errorcluster)  [unwired: 2 in]
            n165 = Cluster To Array(cluster=w239) -> (array=w248:refnum<vi>[])
            n166 = invoke on="Invoke Node" class="VI" method="FP.Open"(reference=w261, error in=w267, "State"=w256) -> (reference out=w260:refnum<vi>, error out=w266:errorcluster)  [unwired: 2 in, 3 out]
            n167 = Delete From Array(array=w248, length=3, index=0) -> (deleted portion=w245:refnum<vi>[], array with subset deleted=w242:refnum<vi>[])
            n168 = call "Module Name--constant.vi"() -> ("Module Name"=w252:string)  [unwired: 11 in]
            n169 = invoke on="Invoke Node" class="VI" method="FP.Center"(reference=w260, error in=w266) -> ()  [unwired: 1 in, 3 out]
            n170 = call "Set Enable State on Multiple Controls.vi"("Enable?"=FALSE, "Controls"=w245) -> ()  [unwired: 10 in]
            n171 = local write "Status"(w250) -> ()
            n172 = call "Module Did Init.vi"("error in (no error)"=w264, "Initialized?"=TRUE, "Origin"=w252) -> ("error out"=w263:errorcluster)  [unwired: 8 in]
            n173 = call "Set Enable State on Multiple Controls.vi"("Enable?"=TRUE, "Controls"=w242) -> ()  [unwired: 10 in]
          }
          frame "---Module Specific---" {
            # "Separator -- The following cases handle messages specific to this Module."
          }
          frame "Load" {
            # "After choosing the file, the tdms file will be loaded"
            n174 = call "MHL_load file.vi"("Data Cluster in"=w272, "error in (no error)"=w274) -> ("Data Cluster out"=w270:T18, "Size (bytes)"=→"Size (bytes)":i64, "error out"=w273:errorcluster)  [unwired: 15 in]
          }
          frame "Update X scale units" {
            # "After choosing the file, the tdms file will be loaded"
            n175 = Variant To Data(error in=w279, type=T4 "micro" ("X Units (micro)"), Variant=w276) -> (data=w275:T4, error out=w278:errorcluster)
            n176 = in-place {
              in-place-border: [w288] -> w282
              in-place-border: w278 -> [w284]
              in-place-border: w275 -> [w285]
              n177 = in-place-cluster #2(w281) -> ("XYgraph Obj"=w287:refnum<class "XYgraph.lvclass">)
              n178 = call-dynamic "Cnvrt X SI units.vi"("reference in"=w287, "X Units (micro)"=w285) -> ("reference out"=w286:refnum<class "XYgraph.lvclass">, "error out"=w283:errorcluster)  [unwired: 16 in]
              n179 = in-place-cluster #2("XYgraph Obj"=w286) -> (w280:T18)
              n180 = Merge Errors(w284, w283) -> (w288:errorcluster)
            }
          }
          frame "Update Y scale units" {
            # "After choosing the file, the tdms file will be loaded"
            n181 = Variant To Data(error in=w293, type=T4 "micro" ("X Units (micro)"), Variant=w290) -> (data=w289:T4, error out=w292:errorcluster)
            n182 = in-place {
              in-place-border: [w302] -> w296
              in-place-border: w292 -> [w301]
              in-place-border: w289 -> [w298]
              n183 = in-place-cluster #3(w295) -> ("XYgraph Obj"=w300:refnum<class "XYgraph.lvclass">)
              n184 = call-dynamic "Cnvrt Y SI units.vi"("reference in"=w300, "Units (micro)"=w298) -> ("reference out"=w299:refnum<class "XYgraph.lvclass">, "error out"=w297:errorcluster)  [unwired: 16 in]
              n185 = in-place-cluster #3("XYgraph Obj"=w299) -> (w294:T18)
              n186 = Merge Errors(w301, w297) -> (w302:errorcluster)
            }
          }
          frame "Stop" {
            # "End user pressed Stop button. Need to request for Acquisition to stop acquiring and for Logger to stop logging."
          }
          frame "Previous file" {
            n187 = call "MHL_previous file.vi"("Delacor_lib_QMH_Message Queue in"=w305, "Data Cluster in"=w307, "error in (no error)"=w309) -> ("Data Cluster out"=w306:T18, "error out"=w308:errorcluster)  [unwired: 15 in]
          }
          frame "Forward file" {
            n188 = call "MHL_forward file.vi"("Delacor_lib_QMH_Message Queue in"=w310, "Data Cluster in"=w312, "error in (no error)"=w314) -> ("Data Cluster out"=w311:T18, "error out"=w313:errorcluster)  [unwired: 15 in]
          }
          frame "Get analysis parameters" {
            # "Gets the analysis parameters"
            n189 = Variant To Data(error in=w322, type=T19 {"Wait Notifier"=refnum, "wait for reply"=FALSE} ("Get analysis parameters Argument"), Variant=w320) -> (data=w318:T19, error out=w321:errorcluster)
            n190 = call "MHL_get analysis parameters.vi"("Data Cluster in"=w316, "Get analysis parameters Argument"=w318, "error in (no error)"=w321) -> ("Data Cluster out"=w315:T18, "error out"=w317:errorcluster)  [unwired: 15 in]
          }
          frame "-------- External Module --------" {
          }
          frame "Filepath updated" {
            # "Update settings of the MAIN gui filepath"
            n191 = Variant To Data(error in=w334, type=T22 {"Settings"={"TDMS Filepath"=path "", "TDMS Directory"=path "", "Dir?"=FALSE}} ("Filepath updated Argument"), Variant=w333) -> (data=w331:T22, error out=w327:errorcluster)
            n192 = Unbundle By Name(w331) -> ("Settings"=w328:T23)
            n193 = call "MHL_file path updated.vi"("Data Cluster in"=w330, "Settings"=w328, "error in (no error)"=w327, "Message Queue in"=w325) -> ("Data Cluster out"=w329:T18, "error out"=w326:errorcluster)  [unwired: 14 in]
          }
          frame "---Copy This Frame---" {
            # "Duplicate this frame when creating new messages.  Change this comment in the duplicated frame to describe this message."
            n194 = Merge Errors(w337) -> (w336:errorcluster)
          }
          frame "Decimate waveforms" {
            # "Duplicate this frame when creating new messages.  Change this comment in the duplicated frame to describe this message."
            n195 = call "MHL_decimate wfms.vi"("Data Cluster in"=w340, "error in (no error)"=w341) -> ("Data Cluster out"=w339:T18, "error out"=w338:errorcluster)  [unwired: 16 in]
          }
          frame "Apply savitzky" {
            # "Duplicate this frame when creating new messages.  Change this comment in the duplicated frame to describe this message."
            n196 = call "MHL_apply Savitzsky.vi"("Data Cluster in"=w343, "error in (no error)"=w344) -> ("Data Cluster out"=w342:T18, "error out"=w345:errorcluster)  [unwired: 16 in]
          }
          frame "Enable Boolean" {
            # "Duplicate this frame when creating new messages.  Change this comment in the duplicated frame to describe this message."
            n197 = Unbundle By Name(w351) -> ("FPref.bools"=w350:T9)
            n198 = Cluster To Array(cluster=w350) -> (array=w349:refnum<vi>[])
            n199 = Array Subset(array=w349, length=1) -> (w347:refnum<vi>[])  [unwired: 1 in]
            n200 = call "Set Enable State on Multiple Controls.vi"("Enable?"=TRUE, "Controls"=w347) -> ()  [unwired: 10 in]
            n201 = Merge Errors(w353) -> (w352:errorcluster)
          }
          frame "---Exit and Error Handling---" {
            # "Separator - The following cases handle errors and exit messages."
          }
          frame "Error" {
            # "Error - Check the error message data and respond accordingly. This message is sent by the \"Error Handler\" VIs at the end of each loop in this application."
            n202 = property on="Property Node" class="Module Admin"(reference=w357) -> ("Accessors:External Launch"=w356:bool)  [unwired: 1 in, 2 out]
            n203 = Variant To Data(error in=w365, type=errorcluster {"status"=FALSE, "code"=0, "source"=""} ("error constant"), Variant=w359) -> (data=w366:errorcluster, error out=w363:errorcluster)
            n204 = call "Error Reported.vi"("Error"=w366) -> ()  [unwired: 10 in, 1 out]
            n205 = case shown="False" w356 {
              tunnel: [w371 _] -> w362
              tunnel: w358 -> [w369 _]
              tunnel: w366 -> [w370 _]
              frame False {
                # "If the module is running standalone, then pop up an error dialog and call the \"Exit\" message."
                n206 = call <vilib>:"Simple Error Handler.vi"("error in (no error)"=w370) -> ()  [unwired: 4 in, 5 out]
                n207 = call-poly <vilib>:"Delacor_lib_QMH_Enqueue Message (poly).vi"("Priority Message? (F)"=TRUE, "Message"="Exit", "Message Queue in"=w369) -> ("error out"=w371:errorcluster)  [unwired: 7 in, 1 out]
              }
              frame True {
                # "If the module was launched externally, calling the Error Reported broadcast VI is the only action performed by the \"Error\" message. The module's caller can then process the error appropriately."
              }
            }
            n208 = Merge Errors(w363, w362) -> (w361:errorcluster)
            n209 = local write "error out"(w361) -> ()
          }
          frame "Exit" {
            w376 = TRUE ("Wait for Module to Stop? (F)")
            w381 = 91  # 91: not all Exit messages will have an argument
            w383 = TRUE  # Stop the VI
            # "DAQ and LOG modules use the settings editor. CML UI module waits for both modules to completely stop before stopping the settings editor."
            # "Release the message queue reference"
            # "Exit - Exit the application."
            n210 = Variant To Data(error in=w390, type=T21 {"Origin"="", "Exit via Stop Module Req?"=FALSE, "Wait for Module to stop?"=FALSE} ("Stop Argument"), Variant=w382) -> (data=w379:T21, error out=w387:errorcluster)
            n211 = call <vilib>:"Clear Errors.vi"("error in (no error)"=w387, "specific error code to clear (0: all)"=w381) -> ("error out"=w389:errorcluster)  [unwired: 4 in, 1 out]
            n212 = control-ref of="This VI"() -> (w378:refnum<vi>)
            n213 = call "Module Name--constant.vi"() -> ("Module Name"=w375:string)  [unwired: 11 in]
            n214 = call "Handle Exit.vi"("Stop Argument"=w379, "Admin in"=w377, "VI reference"=w378) -> ("error out"=w386:errorcluster)  [unwired: 7 in, 1 out]
            n215 = call "Stop Module.vi"("Wait for Module to Stop? (F)"=w376, "Origin"=w375) -> ("error out"=w373:errorcluster)  [unwired: 9 in]
            n216 = call "Stop Module.vi"("Wait for Module to Stop? (F)"=w376, "Origin"=w375) -> ("error out"=w372:errorcluster)  [unwired: 9 in]
            n217 = call-dynamic "Delacor_lib_QMH_Release Message Queue.vi"("error in"=w389, "Message Queue"=w385) -> ("error out"=w388:errorcluster)  [unwired: 9 in]
            n218 = Merge Errors(w373, w372) -> (w391:errorcluster)
            n219 = Merge Errors(w388, w386) -> (w374:errorcluster)
            n220 = call <vilib>:"Clear Errors.vi"("error in (no error)"=w391) -> ("error out"=w392:errorcluster)  [unwired: 5 in, 1 out]
            n221 = call "Stop Module.vi"("error in"=w392, "Wait for Module to Stop? (F)"=w376, "Origin"=w375) -> ()  [unwired: 8 in, 1 out]
          }
          frame Default {
            # "'Default' case only runs if there is a message that isn't defined in any of the other cases.  Output a programming error."
            n222 = call "Module Name--constant.vi"() -> ("Module Name"=w393:string)  [unwired: 11 in]
            n223 = xnode ("Error Ring")("parameter 0"=w394, "parameter 1"=w393) -> ("error out"=w398:errorcluster)
            n224 = Merge Errors(w396, w398) -> (w397:errorcluster)
          }
        }
        n225 = call-dynamic "Delacor_lib_QMH_Error Handler - Message Handling Loop.vi"("error in"=w237, "Message Queue in"=w227) -> ("dup error in"=w234:errorcluster)  [unwired: 8 in, 1 out]
      }
    }
    frame Error {
      w411 = TRUE ("Wait for Module to Stop? (F)")
      # "Synchronize Caller Events.vi will inform Start Module.vi that the module has launched and will let the code calling Start Module.vi register for broadcasts and would permit the caller receive the broadcast that an error occurred at launch time."
      n226 = call-dynamic "Delacor_lib_QMH_Release Message Queue.vi"("error in"=w408, "Message Queue"=w409) -> ("error out"=w407:errorcluster)  [unwired: 9 in]
      n227 = call "Synchronize Caller Events.vi"("Singleton Module Admin in"=w412) -> ("error out"=w417:errorcluster)  [unwired: 9 in, 1 out]
      n228 = call "Module Name--constant.vi"() -> ("Module Name"=w415:string)  [unwired: 11 in]
      n229 = call "Module Name--constant.vi"() -> ("Module Name"=w410:string)  [unwired: 11 in]
      n230 = call "Stop Module.vi"("Wait for Module to Stop? (F)"=w411, "Origin"=w410) -> ()  [unwired: 9 in, 1 out]
      n231 = call "Stop Module.vi"("Wait for Module to Stop? (F)"=w411, "Origin"=w410) -> ()  [unwired: 9 in, 1 out]
      n232 = call "Stop Module.vi"("Wait for Module to Stop? (F)"=w411, "Origin"=w410) -> ()  [unwired: 9 in, 1 out]
      n233 = Format Into String(format string="An error occurred during initialization. %s is no longer running.", w415) -> (resulting string=w413:string)  [unwired: 2 in, 1 out]
      n234 = Merge Errors(w407, w417) -> (w418:errorcluster)
      n235 = call "Error Reported.vi"("Additional Information"=w413, "Error"=w418) -> ()  [unwired: 9 in, 1 out]
    }
  }
  n236 = Merge Errors(w51, w54) -> (w50:errorcluster)
  n237 = call "Close Module.vi"("error in (no error)"=w50, "Module Admin in"=w39) -> ("error out"=w52:errorcluster, "External Launch"=w32:bool, "Module Admin out"=w33:refnum<class "Delacor_lib_QMH_Module Admin.lvclass">)  [unwired: 7 in]
  n238 = Unregister For Events(event registration refnum=w38, error in=w52) -> (error out=w49:errorcluster)
  "error out" <- w49
  n239 = case "External Launch?" shown="True" w32 {
    tunnel: w49 -> [_ w419]
    frame False {
    }
    frame True {
      n240 = case shown="No Error" w419 {
        frame No Error {
          n241 = invoke class="VI" method="FP.Close"() -> ()  [unwired: 3 in, 3 out]
        }
        frame Error {
          n242 = invoke on="Invoke Node" class="VI" method="FP.Open"("Activate"=TRUE ("Activate?")) -> ()  [unwired: 4 in, 5 out]
        }
      }
    }
  }
  n243 = local write "Module Admin"(w33) -> ()
